vi "calculadora.vi"() -> ()   [LabVIEW 2013]
panel:
  out "Numeric 6":dbl
  out "Numeric 4":dbl
  out "Numeric 3":dbl
  out "Numeric 5":dbl
  in  "Numeric 2":dbl
  in  "Numero 1":dbl
  out "Numeric":dbl
  # "UNIVERSIDAD DE CUNDINAMARCA\nINGENIERIA DE SISTEMAS \nELECTIVA PROFECIONAL IV\nANDY LEANDRO CAMARGO"
  # "suma"
  # "resta"
  # "multiplicacion"
  # "divicion"
  # "raiz numero 1"
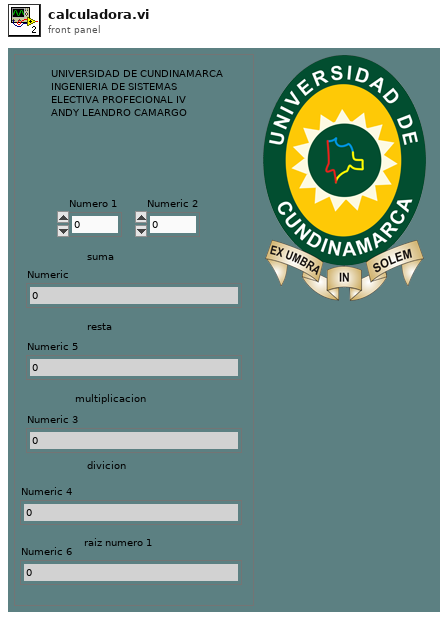
[diagram p1: front panel]
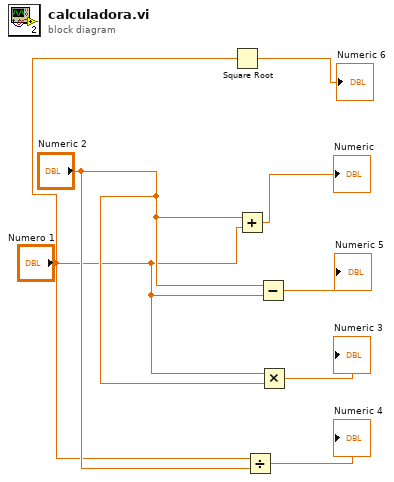
[diagram p0: block diagram]
diagram:
  n1 = Square Root(x="Numero 1") -> (sqrt(x)=→"Numeric 6":dbl)
  n2 = Add(x="Numeric 2", y="Numero 1") -> (x+y=→"Numeric":dbl)
  n3 = Divide(x="Numero 1", y="Numeric 2") -> (x/y=→"Numeric 4":dbl)
  n4 = Subtract(x="Numeric 2", y="Numero 1") -> (x-y=→"Numeric 5":dbl)
  n5 = Multiply(x="Numero 1", y="Numeric 2") -> (x*y=→"Numeric 3":dbl)
